vi "Assert Not In Range.vi"(7 "Message (\"\")":string, 8 "error in (no error)":errorcluster, 9 "Minimum":ext, 10 "Actual":ext, 11 "Maximum":ext) -> (0 "error out":errorcluster)   [LabVIEW 2017, in "Transparent Assertions.lvlib"]
doc: "Asserts that a value is not greater than or equal to the maximum value and not less than or equal to the minimum value. Returns an error if the assertion fails, and optionally appends a custom message to the error."
uses:
  Transparent Assertions.lvlib
  Logical And/Logical And.lvclass
  C:/Users/pasca/Projects/Home/TransparentAssertions/src/Transparent Assertions/Constraints/Binary Operator/Binary Operator.lvclass
  C:/Users/pasca/Projects/Home/TransparentAssertions/src/Transparent Assertions/Constraints/Constraint/Constraint.lvclass
  Logical Or/Logical Or.lvclass
  LogicalNot/LogicalNot.lvclass
  Is Less Than/Is Less Than.lvclass
  IsEqual/IsEqual.lvclass
  Is Greater Than/Is Greater Than.lvclass
  UnaryOperator/UnaryOperator.lvclass
  Binary Operator/Binary Operator.lvclass
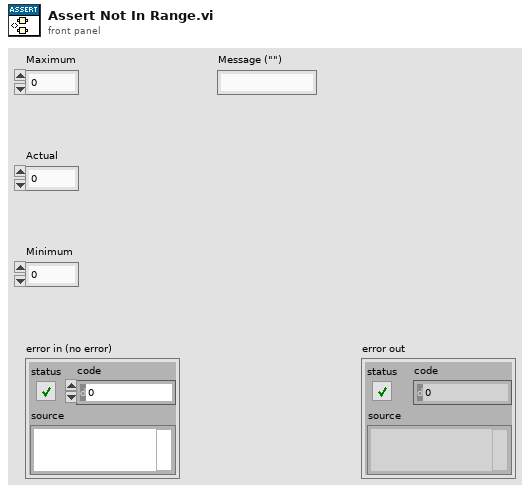
[diagram p1: front panel]
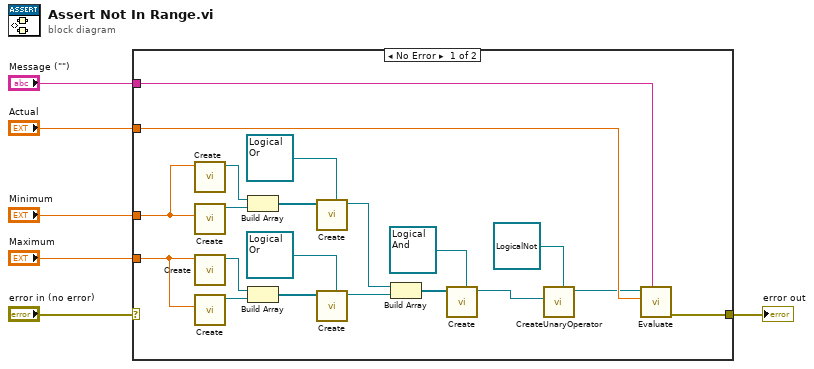
[diagram p0: block diagram]
diagram:
  n1 = case shown="No Error" "error in (no error)" {
    selector: "error in (no error)" -> [_ w27]
    tunnel: "Actual" -> [w26 _]
    tunnel: [w25 w27] -> w6
    tunnel: "Message (\"\")" -> [w24 _]
    tunnel: "Minimum" -> [w23 _]
    tunnel: "Maximum" -> [w22 _]
    frame No Error {
      n2 = call "Create.vi"("Expected"=w23) -> ("Is Greater Than"=w19:refnum<class "Is Greater Than.lvclass">)  [unwired: 9 in, 1 out]
      n3 = call "Create.vi"("Expected"=w23) -> ("IsEqual"=w18:refnum<class "IsEqual.lvclass">)  [unwired: 9 in, 1 out]
      n4 = call "Create.vi"("Expected"=w22) -> ("Is Less Than"=w21:refnum<class "Is Less Than.lvclass">)  [unwired: 9 in, 1 out]
      n5 = call "Create.vi"("Expected"=w22) -> ("IsEqual"=w20:refnum<class "IsEqual.lvclass">)  [unwired: 9 in, 1 out]
      n6 = Build Array(w19, w18) -> (w16:refnum<class "Constraint.lvclass">[])
      n7 = Build Array(w21, w20) -> (w17:refnum<class "Constraint.lvclass">[])
      n8 = call "Create.vi"("Binary Operator in"=refnum<class "Logical Or.lvclass"> refnum ("Transparent Assertions.lvlib:Constraints.lvlib:Logical Or.lvclass"), "Constraints"=w16) -> ("Binary Operator"=w13:refnum<class "Logical Or.lvclass">)  [unwired: 8 in, 1 out]
      n9 = call "Create.vi"("Binary Operator in"=refnum<class "Logical Or.lvclass"> refnum ("Transparent Assertions.lvlib:Constraints.lvlib:Logical Or.lvclass"), "Constraints"=w17) -> ("Binary Operator"=w14:refnum<class "Logical Or.lvclass">)  [unwired: 8 in, 1 out]
      n10 = Build Array(w13, w14) -> (w12:refnum<class "Logical Or.lvclass">[])
      n11 = call "Create.vi"("Binary Operator in"=refnum<class "Logical And.lvclass"> refnum ("Transparent Assertions.lvlib:Constraints.lvlib:Logical And.lvclass"), "Constraints"=w12) -> ("Binary Operator"=w11:refnum<class "Logical And.lvclass">)  [unwired: 8 in, 1 out]
      n12 = call-dynamic "CreateUnaryOperator.vi"("UnaryOperator In"=refnum<class "LogicalNot.lvclass"> refnum ("Transparent Assertions.lvlib:Constraints.lvlib:LogicalNot.lvclass"), "Constraint"=w11) -> ("UnaryOperator"=w8:refnum<class "UnaryOperator.lvclass">)  [unwired: 8 in, 1 out]
      n13 = call-dynamic "Evaluate.vi"("Message (\"\")"=w24, "Actual"=w26, "Constraint in"=w8) -> ("error out"=w25:errorcluster)  [unwired: 7 in, 1 out]
    }
    frame Error {
    }
  }
  "error out" <- w6
